vi "toml_section_names.vi"(8 "error in (no error)":errorcluster, 11 "path in":path) -> (0 "error out":errorcluster, 2 "sections":cluster{"section":string[]}[](array[cluster]), 3 "path out":path)   [LabVIEW 2017]
uses:
  toml_fg_action.ctl
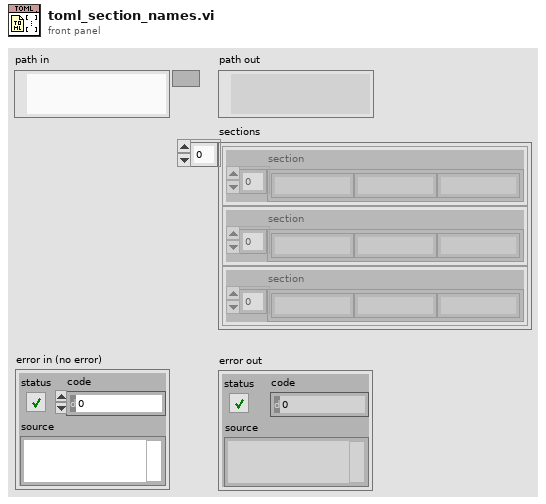
[diagram p1: front panel]
types:
  T1 = typedef "toml_fg_action.ctl" = enum8{"null", "get", "set", "pop", "import", "export", "drop", "sections", "keys", "remove"}
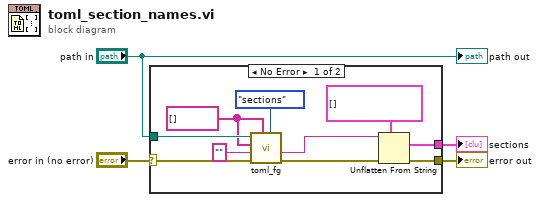
[diagram p0: block diagram]
diagram:
  n1 = case shown="No Error" "error in (no error)" {
    selector: "error in (no error)" -> [w14 w15]
    tunnel: [w10 w15] -> w3
    tunnel: "path in" -> [w13 _]
    tunnel: [w5 _] -> w1
    frame No Error {
      w8 = string[] [] ("section")
      n2 = call "toml_fg.vi"("action"=toml_fg_action."sections", "section"=w8, "error in (no error)"=w14, "value in"="", "key"=w8, "path in"=w13) -> ("error out"=w11:errorcluster, "value out"=w9:string)  [unwired: 2 in, 2 out]
      n3 = Unflatten From String(type=cluster{"section":string[]}[] [] ("sections"), binary string=w9, error in (no error)=w11) -> (value=w5:cluster{"section":string[]}[], error out=w10:errorcluster)  [unwired: 2 in, 1 out]
    }
    frame Error {
    }
  }
  "error out" <- w3
  "sections" <- w1
  "path out" <- "path in"
